vi "Delete csv.vi"() -> ()   [LabVIEW 2022 SP3]
panel:
  in  "Done":bool
  in  "Delete":bool
  out "results":string
  out "Data Folder:":path=path "/Users/crogers/Desktop/Curtin2/Data"
  # "Searching:"
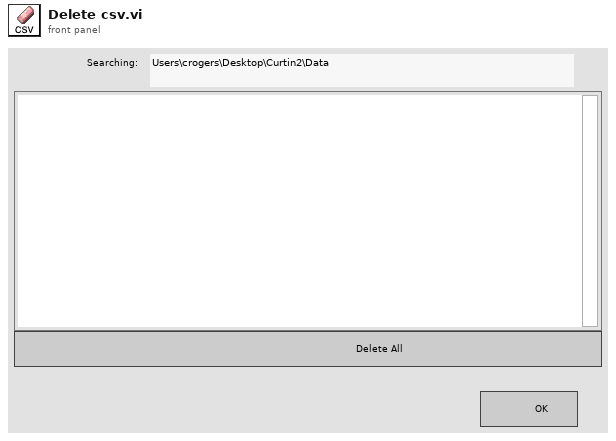
[diagram p1: front panel]
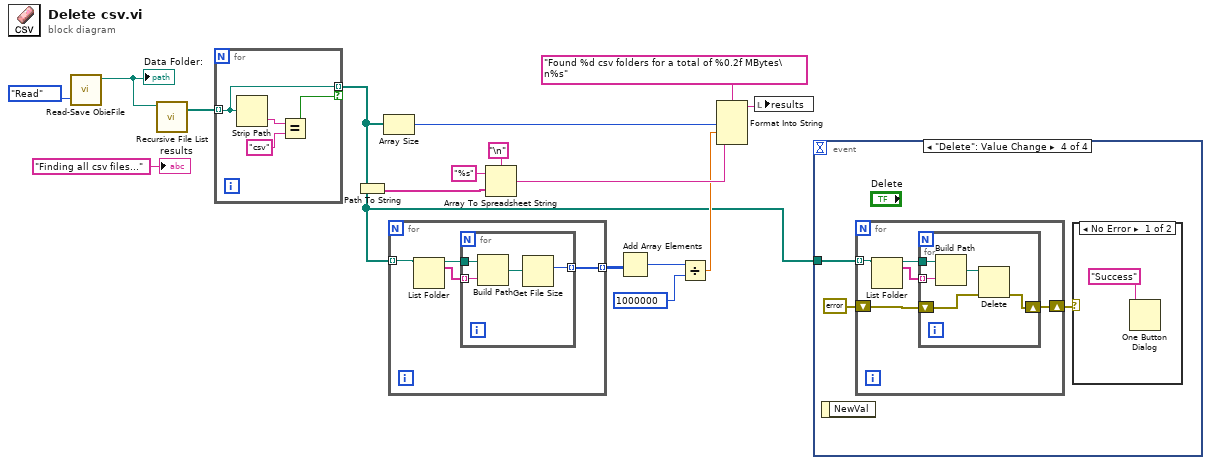
[diagram p0: block diagram]
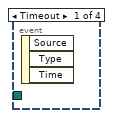
[diagram p2: hidden frame]
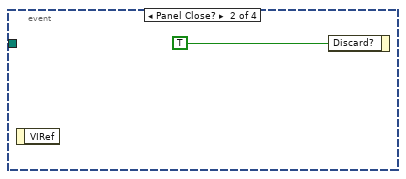
[diagram p3: hidden frame]
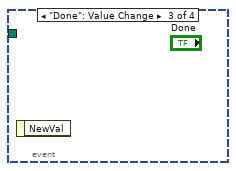
[diagram p4: hidden frame]
diagram:
  n1 = call "Read-Save ObieFile.vi"("Task"=enum16{"Save", "Read"}."Read") -> ("DataPath Out"=w15:path)  [unwired: 8 in, 2 out]
  "Data Folder:" <- w15
  n2 = call <vilib>:"Recursive File List.vi"("Folder Path"=w15) -> ("All Folders"=w14:path[])  [unwired: 6 in, 4 out]
  n3 = for {
    tunnel: w14 -> [w19] mode=indexing
    tunnel: [w19] -> w1 mode=indexing if=w18
    n4 = Strip Path(path=w19) -> (name=w17:string)  [unwired: 1 out]
    n5 = Equal?(x=w17, y="csv") -> (x = y?=w18:bool)
  }
  n6 = Path To String(path=w1) -> (string=w9:string[])
  n7 = Array Size(array=w1) -> (size(s)=w12:i32)
  n8 = for {
    tunnel: w1 -> [w24] mode=indexing
    tunnel: [w21] -> w2 mode=indexing
    n9 = List Folder(path=w24) -> (path out=w23:path, filenames=w22:string[])  [unwired: 3 in, 2 out]
    n10 = for {
      tunnel: w23 -> [w28]
      tunnel: w22 -> [w27] mode=indexing
      tunnel: [w25] -> w21 mode=indexing
      n11 = Build Path(base path=w28, name or relative path=w27) -> (appended path=w26:path)
      n12 = Get File Size(file=w26) -> (size (in bytes)=w25:i64)  [unwired: 1 in, 2 out]
    }
  }
  n13 = Array To Spreadsheet String(delimiter (Tab)="\n", array=w9, 3:"%s" ("format string")) -> (spreadsheet string=w6:string)
  n14 = Add Array Elements(numeric array=w2) -> (sum=w5:i64)
  n15 = Divide(x=w5, y=i64 1000000) -> (x/y=w4:dbl)
  n16 = Format Into String(format string="Found %d csv folders for a total of %0.2f MBytes\n%s", w12, w4, w6) -> (resulting string=w10:string)  [unwired: 2 in, 1 out]
  n17 = local write "results"(w10) -> ()
  n18 = event shown="[3] \"Delete\": Value Change" {
    selector: _ -> [_ _ _ _]
    dyn-events: _ -> [_ _ _ _]
    timeout: _ -> [_ _ _ _]
    tunnel: w1 -> [_ _ _ w32]
    event Timeout {
      n19 = event-data() -> ()  [unwired: 1 in, 3 out]
    }
    event Panel Close? {
      n20 = event-data() -> ()  [unwired: 1 in, 1 out]
      n21 = event-data("Discard?"=TRUE) -> ()  [unwired: 1 in, 1 out]
    }
    event "Done": Value Change {
      n22 = event-data() -> ()  [unwired: 1 in, 1 out]
    }
    event "Delete": Value Change {
      n23 = event-data() -> ()  [unwired: 1 in, 1 out]
      n24 = for {
        tunnel: w32 -> [w38] mode=indexing
        shift-right: [w34] -> w30
        shift-left: errorcluster {"status"=FALSE, "code"=0, "source"=""} ("error out") -> [w35]
        n25 = List Folder(path=w38) -> (path out=w37:path, filenames=w36:string[])  [unwired: 3 in, 2 out]
        n26 = for {
          tunnel: w37 -> [w43]
          tunnel: w36 -> [w42] mode=indexing
          shift-right: [w40] -> w34
          shift-left: w35 -> [w39]
          n27 = Build Path(base path=w43, name or relative path=w42) -> (appended path=w41:path)
          n28 = Delete(path (use dialog)=w41, error in=w39) -> (error out=w40:errorcluster)  [unwired: 3 in, 2 out]
        }
      }
      n29 = case shown="No Error" w30 {
        frame No Error {
          n30 = One Button Dialog(message="Success") -> ()  [unwired: 1 in, 1 out]
        }
        frame Error {
        }
      }
    }
  }
  "results" <- "Finding all csv files..." ("task")
